vi "Read Rows.vi"(8 "error in (no error)":errorcluster, 11 "Config-Sqlite in":refnum<class "Config-Sqlite.lvclass">) -> (0 "error out":errorcluster, 2 "Configs":map{i32, T1}(c390), 3 "Config-Sqlite out":refnum<class "Config-Sqlite.lvclass">)   [LabVIEW 2020, in "CDM-Config.lvlib" / "Config-Sqlite.lvclass"]
uses:
  Config-Sqlite.lvclass
  Config.ctl
  Meta Data.ctl
  Config-Sqlite.lvclass/Config-Sqlite.ctl
  <vilib>/drjdpowell/SQLite Library/SQL Statement/SQL Statement.lvclass/SQL Statement.ctl
  <vilib>/drjdpowell/SQLite Library/SQL Statement/Column I64.vi
  <vilib>/drjdpowell/SQLite Library/SQL Statement/Error Message.vi
  <vilib>/drjdpowell/SQLite Library/SQL Statement/Column String.vi
  <vilib>/drjdpowell/SQLite Library/SQL Connection/Connection.lvclass
  <vilib>/drjdpowell/SQLite Library/SQL Statement/SQL Statement.lvclass
  CDM-Config.lvlib
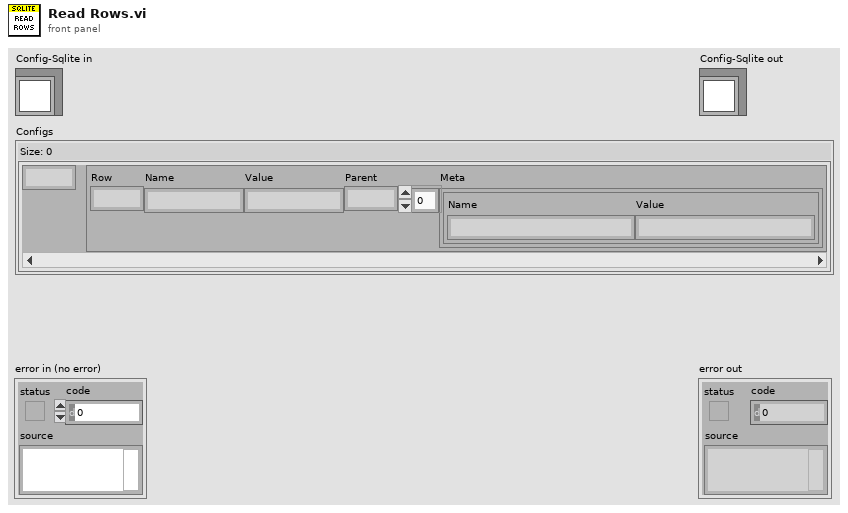
[diagram p1: front panel]
types:
  T1 = typedef "CDM-Config.lvlib/Config-Sqlite.lvclass/Config.ctl" = cluster{"Row":i32, "Name":string, "Value":string, "Parent":i32, "Meta":T2[]}
  T2 = typedef "CDM-Config.lvlib/Meta Data.ctl" = cluster{"Name":string, "Value":string}
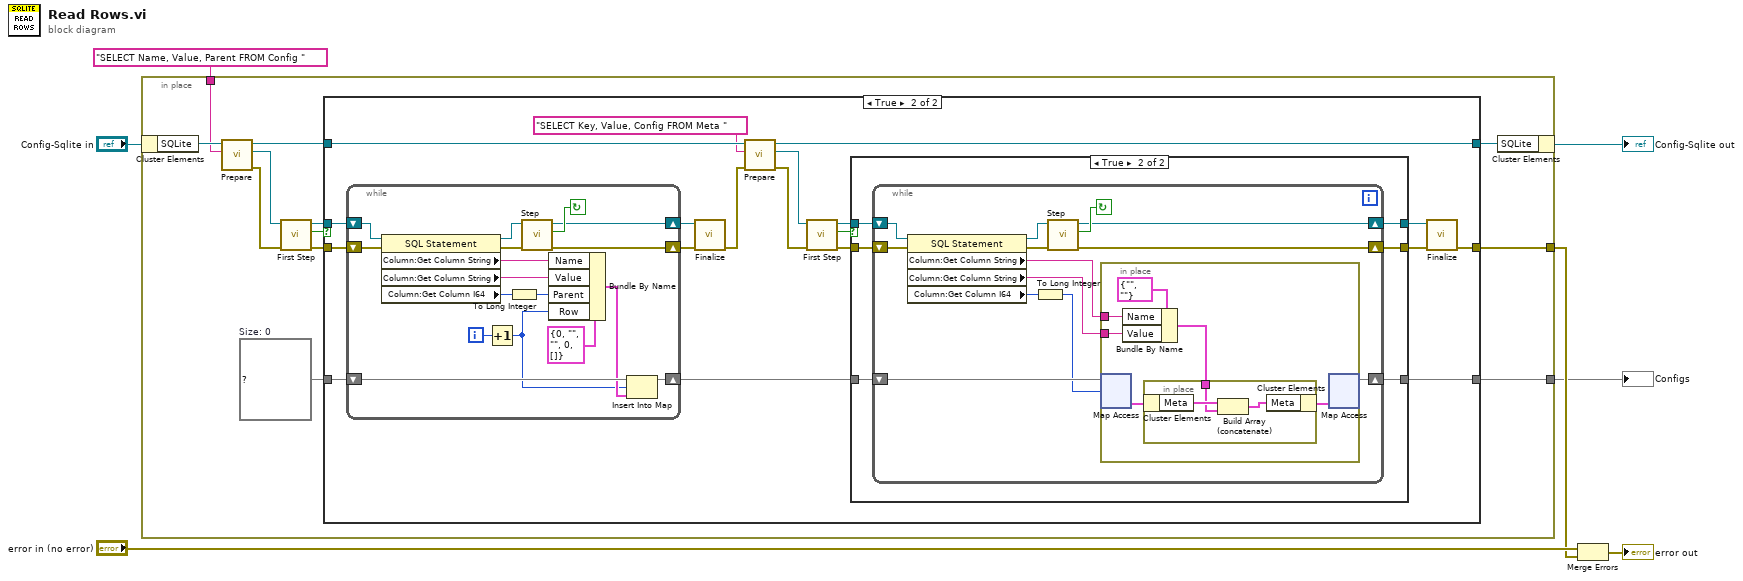
[diagram p0: block diagram]
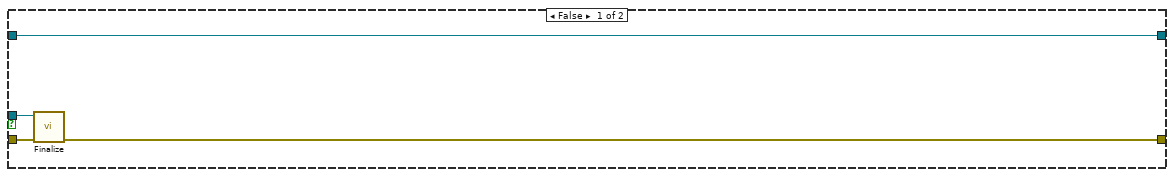
[diagram p2: hidden frame]
diagram:
  n1 = in-place {
    in-place-border: "SELECT Name, Value, Parent FROM Config " -> [w18]
    in-place-border: [w9] -> w2
    in-place-border: [w8] -> w1
    w12 = map{i32, T1} {}  # Size: 0
    n2 = in-place-cluster #1("Config-Sqlite in") -> ("SQLite"=w19:refnum<class "Connection.lvclass">)
    n3 = call <vilib>:"Prepare.vi"("SQL"=w18, "SQLite Connection in"=w19) -> ("error out"=w16:errorcluster, "SQL Statement"=w17:refnum<class "SQL Statement.lvclass">, "SQLite Connection"=w11:refnum<class "Connection.lvclass">)  [unwired: 5 in, 2 out]
    n4 = call <vilib>:"First Step.vi"("error in (no error)"=w16, "SQL Statement in"=w17) -> ("error out"=w14:errorcluster, "Row returned"=w15:bool, "SQL Statement"=w13:refnum<class "SQL Statement.lvclass">)  [unwired: 7 in]
    n5 = case shown="True" w15 {
      tunnel: w14 -> [w23 w41]
      tunnel: w13 -> [w22 w42]
      tunnel: w12 -> [_ w38]
      tunnel: w11 -> [w21 w37]
      tunnel: [w21 w29] -> w10
      tunnel: [w20 w25] -> w9
      tunnel: [_ w24] -> w8
      frame False {
        n6 = call <vilib>:"Finalize.vi"("error in (no error)"=w23, "SQL Statement in"=w22) -> ("error out"=w20:errorcluster)  [unwired: 9 in]
      }
      frame True {
        n7 = while {
          shift-right: [w54] -> w40
          shift-left: w42 -> [w58]
          shift-right: [w53] -> w39
          shift-left: w41 -> [w59]
          shift-right: [w43] -> w28
          shift-left: w38 -> [w46]
          i -> [w52]
          stop <- w55 continue-if-true
          n8 = property on="Extract Column Data" class="SQL Statement"(reference=w58, error in=w59) -> (reference out=w56:refnum<class "SQL Statement.lvclass">, error out=w57:errorcluster, "Column:Get Column String"=w49:string, "Column:Get Column String"=w48:string, "Column:Get Column I64"=w51:i64)
          n9 = Increment(x=w52) -> (x+1=w44:i32)
          n10 = To Long Integer(number=w51) -> (32bit integer=w47:i32)
          n11 = call <vilib>:"Step.vi"("error in (no error)"=w57, "SQL Statement in"=w56) -> ("error out"=w53:errorcluster, "Row returned"=w55:bool, "SQL Statement"=w54:refnum<class "SQL Statement.lvclass">)  [unwired: 7 in]
          n12 = Bundle By Name(cluster=T1 {"Row"=0, "Name"="", "Value"="", "Parent"=0, "Meta"=[]} ("Config Row"), "Name"=w49, "Value"=w48, "Parent"=w47, "Row"=w44) -> (w45:T1)
          n13 = Insert Into Map(map in=w46, key=w44, value=w45) -> (map out=w43:map{i32, T1})  [unwired: 2 out]
        }
        n14 = call <vilib>:"Finalize.vi"("error in (no error)"=w39, "SQL Statement in"=w40) -> ("error out"=w36:errorcluster)  [unwired: 9 in]
        n15 = call <vilib>:"Prepare.vi"("error in (no error)"=w36, "SQL"="SELECT Key, Value, Config FROM Meta ", "SQLite Connection in"=w37) -> ("error out"=w33:errorcluster, "SQL Statement"=w34:refnum<class "SQL Statement.lvclass">, "SQLite Connection"=w29:refnum<class "Connection.lvclass">)  [unwired: 4 in, 2 out]
        n16 = call <vilib>:"First Step.vi"("error in (no error)"=w33, "SQL Statement in"=w34) -> ("error out"=w31:errorcluster, "Row returned"=w32:bool, "SQL Statement"=w30:refnum<class "SQL Statement.lvclass">)  [unwired: 7 in]
        n17 = case shown="True" w32 {
          tunnel: w31 -> [w61 w67]
          tunnel: w30 -> [w62 w68]
          tunnel: w28 -> [w60 w66]
          tunnel: [w62 w65] -> w26
          tunnel: [w61 w64] -> w27
          tunnel: [w60 w63] -> w24
          frame False {
          }
          frame True {
            n18 = while {
              shift-right: [w76] -> w65
              shift-left: w68 -> [w80]
              shift-right: [w75] -> w64
              shift-left: w67 -> [w81]
              shift-right: [w73] -> w63
              shift-left: w66 -> [w74]
              stop <- w77 continue-if-true
              n19 = property on="Extract Column Data" class="SQL Statement"(reference=w80, error in=w81) -> (reference out=w78:refnum<class "SQL Statement.lvclass">, error out=w79:errorcluster, "Column:Get Column String"=w69:string, "Column:Get Column String"=w70:string, "Column:Get Column I64"=w72:i64)
              n20 = To Long Integer(number=w72) -> (32bit integer=w71:i32)
              n21 = call <vilib>:"Step.vi"("error in (no error)"=w79, "SQL Statement in"=w78) -> ("error out"=w75:errorcluster, "Row returned"=w77:bool, "SQL Statement"=w76:refnum<class "SQL Statement.lvclass">)  [unwired: 7 in]
              n22 = in-place {
                in-place-border: w70 -> [w83]
                in-place-border: w69 -> [w84]
                n23 = in-place-map #2(w74, w71) -> (w87:T1)  [unwired: 1 in, 1 out]
                n24 = Bundle By Name(cluster=T2 {"Name"="", "Value"=""} ("Meta Data"), "Name"=w84, "Value"=w83) -> (w82:T2)
                n25 = in-place {
                  in-place-border: w82 -> [w88]
                  n26 = in-place-cluster #3(w87) -> ("Meta"=w90:T2[])
                  n27 = Build Array (concatenate)(w90, w88) -> (w89:T2[])
                  n28 = in-place-cluster #3("Meta"=w89) -> (w86:T1)
                }
                n29 = in-place-map #2(w86) -> (w73:map{i32, T1})  [unwired: 1 in, 2 out]
              }
            }
          }
        }
        n30 = call <vilib>:"Finalize.vi"("error in (no error)"=w27, "SQL Statement in"=w26) -> ("error out"=w25:errorcluster)  [unwired: 9 in]
      }
    }
    n31 = in-place-cluster #1("SQLite"=w10) -> (→"Config-Sqlite out":refnum<class "Config-Sqlite.lvclass">)
  }
  "Configs" <- w1
  n32 = Merge Errors("error in (no error)", w2) -> (→"error out":errorcluster)
